vi "Populate Tables From Document.vi"(8 "error in (no error)":errorcluster, 11 "xwpfDocument in":refnum<class "xwpfDocument.lvclass">) -> (0 "error out":errorcluster, 3 "xwpfDocument out":refnum<class "xwpfDocument.lvclass">)   [LabVIEW 2017, in "Word_Specific.lvlib" / "xwpfDocument.lvclass"]
uses:
  xwpfDocument.lvclass
  xwpfDocument.lvclass/xwpfDocument.ctl
  C:/Users/Neo/Desktop/Dev_Tools_BR/LabVIEW_NPOI/lib/NPOI 2.1.1/NPOI.OOXML.dll
  lib/NPOI 2.1.1/NPOI.OOXML.dll
  xwpfTable/xwpfTable.lvclass
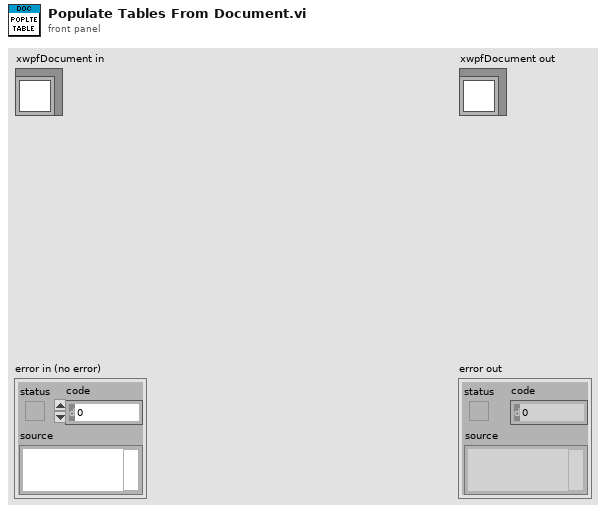
[diagram p1: front panel]
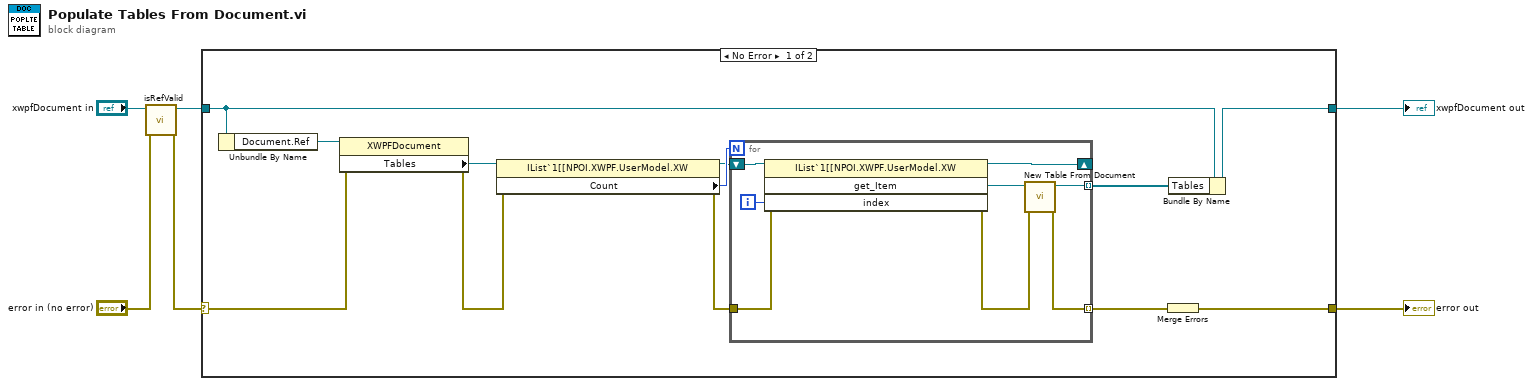
[diagram p0: block diagram]
diagram:
  n1 = call-dynamic "isRefValid.vi"("error in (no error)"="error in (no error)", "xwpfDocument in"="xwpfDocument in") -> ("error out"=w1:errorcluster, "xwpfDocument out"=w3:refnum<class "xwpfDocument.lvclass">)  [unwired: 8 in]
  n2 = case shown="No Error" w1 {
    selector: w1 -> [w14 w28]
    tunnel: [w8 w28] -> w6
    tunnel: [w10 w27] -> w4
    tunnel: w3 -> [w11 w27]
    frame No Error {
      n3 = Unbundle By Name(w11) -> ("Document.Ref"=w9:refnum<k24>)
      n4 = property class="XWPFDocument"(reference=w9, error in=w14) -> (error out=w15:errorcluster, "Tables"=w18:refnum<k24>)  [unwired: 1 out]
      n5 = property class="IList`1[[NPOI.XWPF.UserModel.XW"(reference=w18, error in=w15) -> (reference out=w7:refnum<k24>, error out=w16:errorcluster, "Count"=w17:i32)
      n6 = for {
        N: w17 -> [_]
        shift-right: [w25] -> _
        shift-left: w7 -> [w26]
        tunnel: [w24] -> w12 mode=indexing
        tunnel: w16 -> [w22]
        tunnel: [w21] -> w13 mode=indexing
        i -> [w19]
        n7 = invoke class="IList`1[[NPOI.XWPF.UserModel.XW" method="get_Item"(reference=w26, error in=w22, "index"=w19) -> (reference out=w25:refnum<k24>, error out=w23:errorcluster, "get_Item"=w20:refnum<k24>)  [unwired: 1 in, 1 out]
        n8 = call "New Table From Document.vi"("error in (no error)"=w23, "Table Ref"=w20) -> ("error out"=w21:errorcluster, "xwpfTable out"=w24:refnum<class "xwpfTable.lvclass">)  [unwired: 8 in]
      }
      n9 = Merge Errors(w13) -> (w8:errorcluster)
      n10 = Bundle By Name(cluster=w11, "Tables"=w12) -> (w10:refnum<class "xwpfDocument.lvclass">)
    }
    frame Error {
    }
  }
  "error out" <- w6
  "xwpfDocument out" <- w4
